vi "Read Audio File Test.vi"(7 "Stop Button":bool, 8 "error in":errorcluster, 11 "Audio File":string="Gotye - Somebody That I Used To Know.mp3") -> (0 "error out":errorcluster, 3 "Read Audio File":dbl(graph))   [LabVIEW 2019]
doc: "This is a test VI to check that an audio file was transferred correctly."
panel:
  # "Reading an Audio File on the NI ELVIS III"
  # "This is a test VI to check that an audio file was transferred correctly."
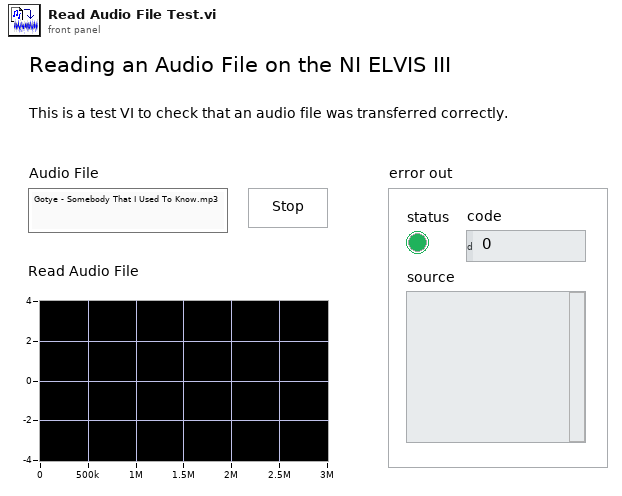
[diagram p1: front panel]
types:
  T1 = enum16{"open", "replace", "create", "open or create", "replace or create", "replace or create with confirmation"}
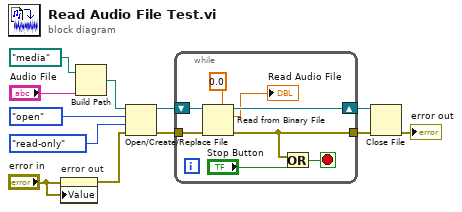
[diagram p0: block diagram]
diagram:
  n1 = property on="error out" class="Clust (strict)"(error in="error in", "Value"="error in") -> (error out=w2:errorcluster)  [unwired: 1 in, 1 out]
  n2 = Build Path(base path=path "/media", name or relative path="Audio File") -> (appended path=w5:path)
  n3 = Open/Create/Replace File(file path (use dialog)=w5, error in=w2, operation (0:open)=T1."open", access (0:read/write)=enum16{"read/write", "read-only", "write-only"}."read-only") -> (refnum out=w9:refnum<file>, error out=w12:errorcluster)  [unwired: 2 in, 1 out]
  n4 = while {
    shift-right: [w19] -> w10
    shift-left: w9 -> [w18]
    tunnel: w12 -> [w20]
    tunnel: [w15] -> w11
    stop <- w14 stop-if-true
    n5 = Read from Binary File(5:0.0, 8:w20, 11:w18) -> (0:w15:errorcluster, 2:→"Read Audio File":dbl, 3:w19:refnum<file>)  [unwired: 3 in, 1 out]
    n6 = Or(x=w15, y="Stop Button") -> (x .or. y?=w14:bool)
  }
  n7 = Close File(refnum=w10, error in=w11) -> (error out=→"error out":errorcluster)  [unwired: 1 out]
